vi "Destroy.vi"(0 "reference in":refnum<class "Generic Utilities.lvclass">, 5 "error in (no error)":errorcluster) -> (14 "reference out":refnum<class "Generic Utilities.lvclass">, 19 "error out":errorcluster)   [LabVIEW 2022 SP3, in "Generic Utilities.lvclass"]
doc: "Destructor."
uses:
  Generic Utilities.lvclass
  <vilib>/addons/_AddQ/G#Object/G#Object.lvclass
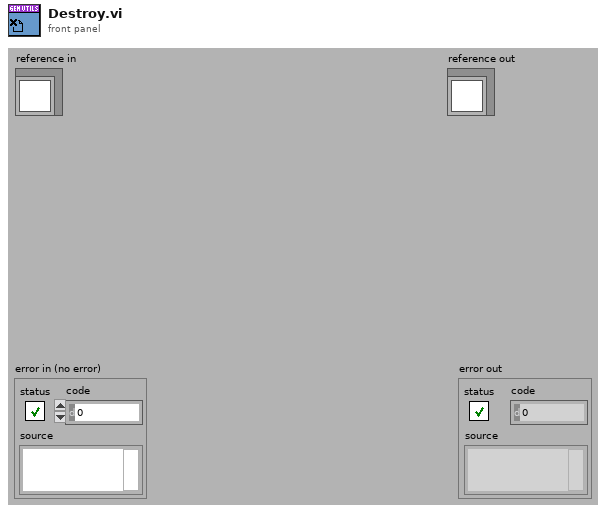
[diagram p1: front panel]
types:
  T1 = typedef "Generic Utilities.lvclass/ObjectAttributes.ctl" = cluster{"GUI Parameters":T2, "State Machine Control":cluster{"Timeout":i32, "State Queue":string[], "State History":string[], "State History Length":i32}, "Logging File Path":path, "OBJ not a refnum?":bool, "Timer Start":timestamp, "FP Refnums":T3}
  T2 = typedef "Generic Utilities.lvclass/GUI Parameters.ctl" = cluster{"Application Name":string, "GUI VI Ref":refnum<vi>, "Close Panel?":bool, "Message Window ref":refnum<vi>, "Version #":string}
  T3 = typedef "Generic Utilities.lvclass/FP Refnums.ctl" = cluster{"Panel refnum":refnum<vi>, "Control Labels":string[], "Refnums":refnum<vi>[]}
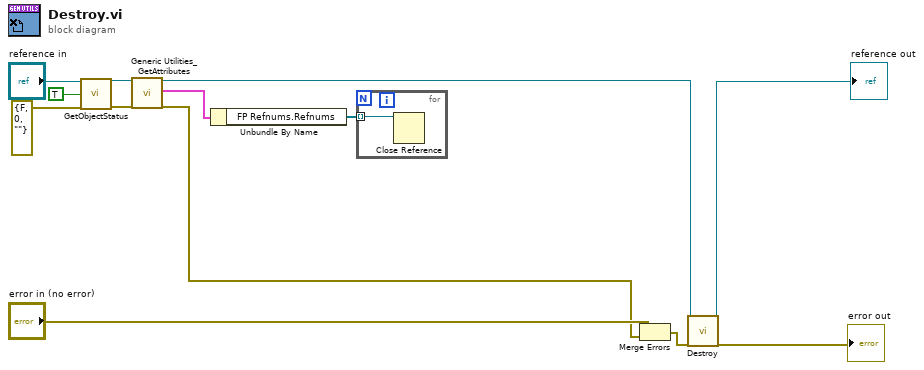
[diagram p0: block diagram]
diagram:
  n1 = call-dynamic "GetObjectStatus.vi"("reference in"="reference in", "simple info (F)"=TRUE ("simple info"), "error in (no error)"=errorcluster {"status"=FALSE, "code"=0, "source"=""}) -> ("reference out"=w6:refnum<class "Generic Utilities.lvclass">, "error out"=w7:errorcluster)  [unwired: 5 in, 10 out]
  n2 = call "Generic Utilities_GetAttributes.vi"("reference in"=w6, "error in (no error)"=w7) -> ("reference out"=w5:refnum<class "Generic Utilities.lvclass">, "attributes"=w4:T1, "error out"=w8:errorcluster)  [unwired: 14 in, 1 out]
  n3 = Unbundle By Name(w4) -> ("FP Refnums.Refnums"=w1:refnum<vi>[])
  n4 = for {
    tunnel: w1 -> [w14] mode=indexing
    n5 = Close Reference(reference=w14) -> ()  [unwired: 1 in, 1 out]
  }
  n6 = Merge Errors("error in (no error)", w8) -> (w12:errorcluster)
  n7 = call-parent "Destroy.vi"("reference in"=w5, "error in (no error)"=w12) -> ("reference out"=→"reference out":refnum<class "Generic Utilities.lvclass">, "error out"=→"error out":errorcluster)  [unwired: 16 in]
